vi "360final.vi"() -> ()   [LabVIEW 2020]
uses:
  <vilib>/Instr/_visa.llb/VISA Configure Serial Port (Instr).vi
panel:
  out "Humidity":dbl(graph)
  out "Thermometer":dbl(graph)
  in  "VISA resource name":refnum<visa-resource-name>
  out "Humidity":dbl(knob) scale=0.0..100.0
  out "Thermometer":dbl(slide) scale=0.0..100.0
  out "GAS Leakage":bool
  in  "Servo":bool
  in  "DC motor":bool
  out "Human Presence":bool
  in  "Light":bool
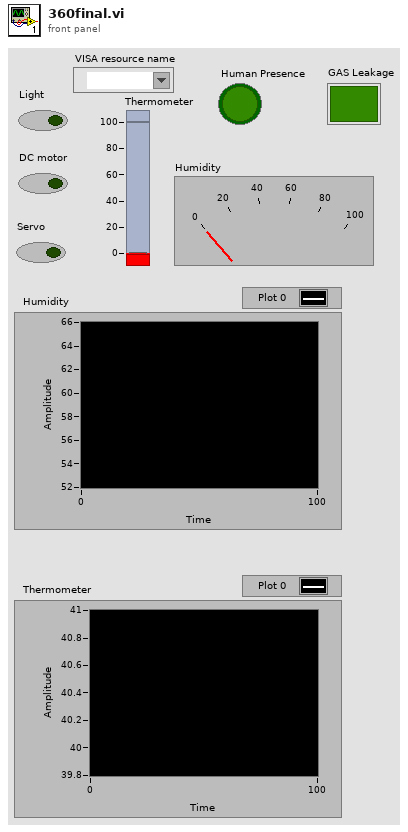
[diagram p1: front panel]
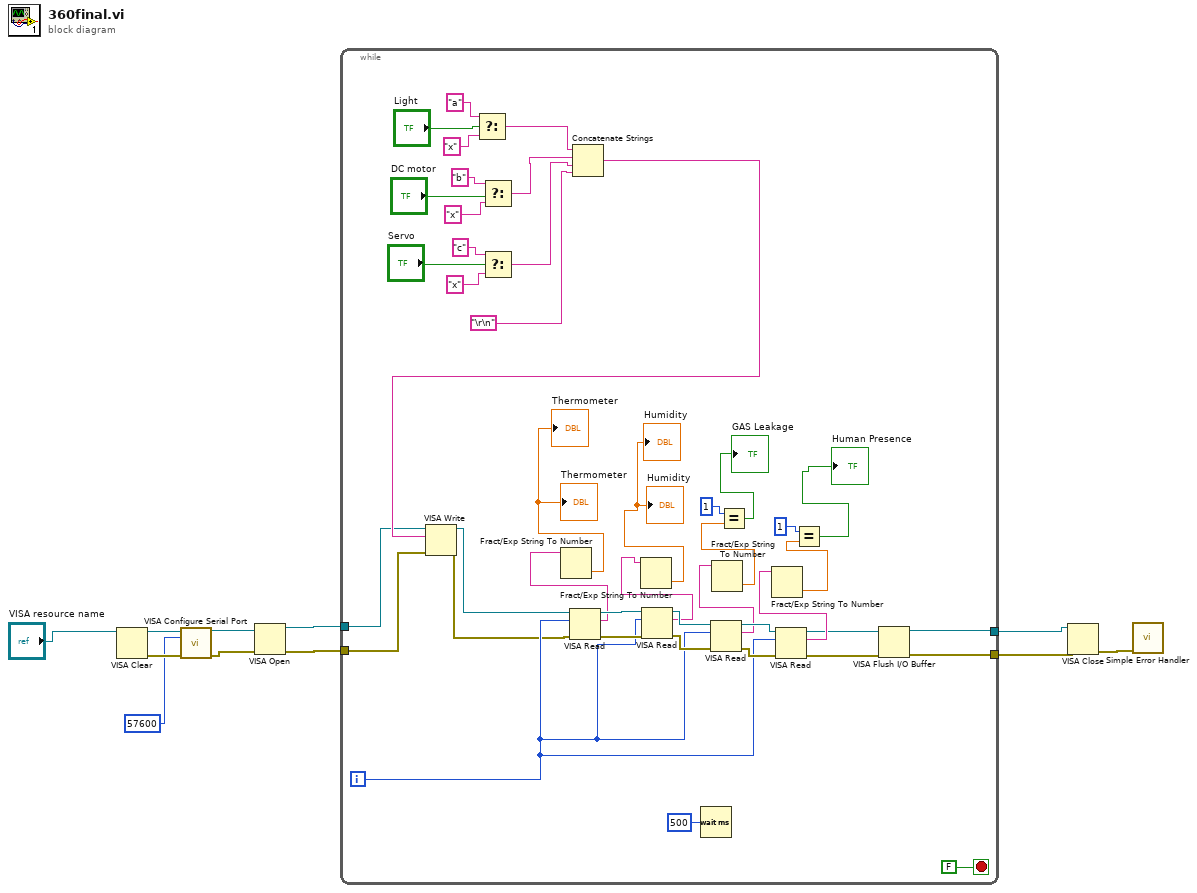
[diagram p0: block diagram]
diagram:
  n1 = VISA Clear(VISA resource name="VISA resource name") -> (VISA resource name out=w4:refnum<visa-resource-name>, error out=w3:errorcluster)  [unwired: 1 in]
  n2 = call-poly "VISA Configure Serial Port"("VISA resource name"=w4, "baud rate (9600)"=u32 57600, "error in (no error)"=w3) -> ("VISA resource name out"=w8:refnum<visa-resource-name>, "error out"=w7:errorcluster)  [unwired: 11 in]
  n3 = VISA Open(error in (no error)=w7, VISA resource name=w8) -> (VISA resource name=w10:refnum<visa-resource-name>, error out=w9:errorcluster)  [unwired: 3 in]
  n4 = while {
    tunnel: w10 -> [w18]
    tunnel: w9 -> [w17]
    tunnel: [w37] -> w6
    tunnel: [w36] -> w5
    i -> [w48]
    stop <- FALSE stop-if-true
    n5 = Select(t="a", s="Light", f="x") -> (s? t:f=w26:string)
    n6 = Select(t="b", s="DC motor", f="x") -> (s? t:f=w25:string)
    n7 = Select(t="c", s="Servo", f="x") -> (s? t:f=w24:string)
    n8 = Concatenate Strings(w26, w25, w24, "\r\n") -> (w19:string)
    n9 = VISA Write(VISA resource name=w18, write buffer=w19, error in (no error)=w17) -> (VISA resource name out=w16:refnum<visa-resource-name>, error out=w15:errorcluster)  [unwired: 1 out]
    n10 = VISA Read(VISA resource name=w16, byte count=w48, error in (no error)=w15) -> (VISA resource name out=w54:refnum<visa-resource-name>, read buffer=w46:string, error out=w53:errorcluster)  [unwired: 1 out]
    n11 = Fract/Exp String To Number(string=w46) -> (number=→"Thermometer" →"Thermometer":dbl)  [unwired: 3 in, 1 out]
    n12 = VISA Read(VISA resource name=w54, byte count=w48, error in (no error)=w53) -> (VISA resource name out=w52:refnum<visa-resource-name>, read buffer=w44:string, error out=w51:errorcluster)  [unwired: 1 out]
    n13 = Fract/Exp String To Number(string=w44) -> (number=→"Humidity" →"Humidity":dbl)  [unwired: 3 in, 1 out]
    n14 = Wait (ms)(milliseconds to wait=u32 500) -> ()  [unwired: 1 out]
    n15 = VISA Read(VISA resource name=w52, byte count=w48, error in (no error)=w51) -> (VISA resource name out=w50:refnum<visa-resource-name>, read buffer=w43:string, error out=w49:errorcluster)  [unwired: 1 out]
    n16 = Fract/Exp String To Number(string=w43) -> (number=w41:dbl)  [unwired: 3 in, 1 out]
    n17 = Equal?(x=1, y=w41) -> (x = y?=→"GAS Leakage":bool)
    n18 = VISA Read(VISA resource name=w50, byte count=w48, error in (no error)=w49) -> (VISA resource name out=w14:refnum<visa-resource-name>, read buffer=w42:string, error out=w13:errorcluster)  [unwired: 1 out]
    n19 = Fract/Exp String To Number(string=w42) -> (number=w40:dbl)  [unwired: 3 in, 1 out]
    n20 = Equal?(x=1, y=w40) -> (x = y?=→"Human Presence":bool)
    n21 = VISA Flush I/O Buffer(VISA resource name=w14, error in (no error)=w13) -> (VISA resource name out=w37:refnum<visa-resource-name>, error out=w36:errorcluster)  [unwired: 1 in]
  }
  n22 = VISA Close(VISA resource name=w6, error in (no error)=w5) -> (error out=w11:errorcluster)
  n23 = call <vilib>:"Simple Error Handler.vi"("error in (no error)"=w11) -> ()  [unwired: 4 in, 5 out]
